vi "Read.vi"(6 "timeout ms (5000)":i32=5000, 8 "error in (no error)":errorcluster, 9 "bytes to read":i32=1024, 11 "LibreVNA in":refnum<class "LibreVNA.lvclass">) -> (0 "error out":errorcluster, 1 "TimeStamp":timestamp, 2 "Recv Buffer":string, 3 "LibreVNA out":refnum<class "LibreVNA.lvclass">)   [LabVIEW 2023, in "LibreVNA.lvclass"]
uses:
  LibreVNA.lvclass
  LibreVNA.lvclass/LibreVNA.ctl
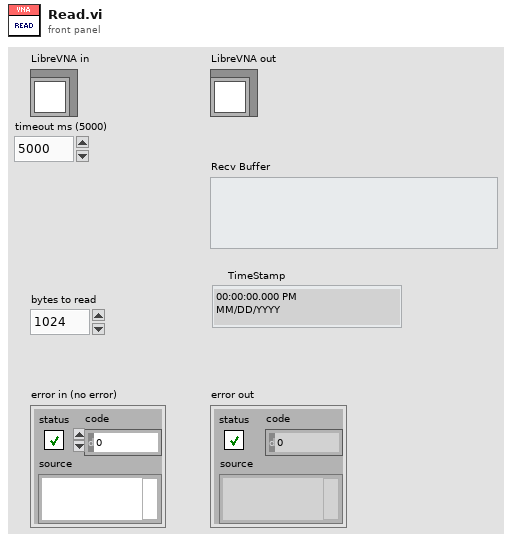
[diagram p1: front panel]
types:
  T1 = enum16{"Standard", "Buffered", "CRLF", "Immediate"}
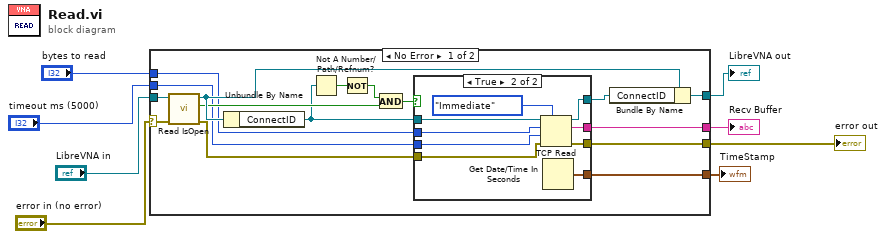
[diagram p0: block diagram]
diagram:
  n1 = case shown="No Error" "error in (no error)" {
    selector: "error in (no error)" -> [w19 w37]
    tunnel: [w14 w37] -> w7
    tunnel: [w16 w36] -> w5
    tunnel: "LibreVNA in" -> [w24 w36]
    tunnel: [w12 _] -> w4
    tunnel: "bytes to read" -> [w11 _]
    tunnel: "timeout ms (5000)" -> [w10 _]
    tunnel: [w9 _] -> w1
    frame No Error {
      n2 = call-dynamic "Read IsOpen.vi"("error in (no error)"=w19, "LibreVNA in"=w24) -> ("error out"=w17:errorcluster, "IsOpen"=w20:bool, "LibreVNA out"=w23:refnum<class "LibreVNA.lvclass">)  [unwired: 7 in]
      n3 = Unbundle By Name(w23) -> ("ConnectID"=w18:refnum<k5>)
      n4 = Not A Number/Path/Refnum?(number/path/refnum=w18) -> (NaN/Path/Refnum?=w22:bool)
      n5 = Not(x=w22) -> (.not. x?=w21:bool)
      n6 = And(x=w21, y=w20) -> (x .and. y?=w13:bool)
      n7 = case shown="True" w13 {
        tunnel: w18 -> [w26 w35]
        tunnel: w17 -> [w25 w34]
        tunnel: [w26 w33] -> w15
        tunnel: [w25 w31] -> w14
        tunnel: [_ w32] -> w12
        tunnel: w11 -> [_ w30]
        tunnel: w10 -> [_ w28]
        tunnel: [_ w27] -> w9
        frame False {
        }
        frame True {
          n8 = TCP Read(connection ID=w35, bytes to read=w30, error in (no error)=w34, 7:T1."Immediate" ("mode (standard)"), 9:w28) -> (connection ID out=w33:refnum<k5>, data out=w32:string, error out=w31:errorcluster)
          n9 = Get Date/Time In Seconds() -> (seconds since 1Jan1904=w27:timestamp)
        }
      }
      n10 = Bundle By Name(cluster=w23, "ConnectID"=w15) -> (w16:refnum<class "LibreVNA.lvclass">)
    }
    frame Error {
    }
  }
  "error out" <- w7
  "LibreVNA out" <- w5
  "Recv Buffer" <- w4
  "TimeStamp" <- w1
